vi "Analyze Target.vi"(10 "Goal Pickiness":T1, 11 "Relevant Data":T2[](array[typedef])) -> (3 "What to do":string)   [LabVIEW 2015]
uses:
  References/Relevant Data.ctl
panel:
  in  "Goal Area":dbl
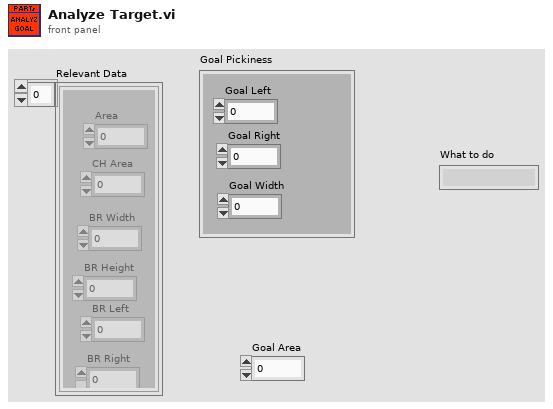
[diagram p1: front panel]
types:
  T1 = cluster{"Goal Left":dbl, "Goal Right":dbl, "Goal Width":dbl}
  T2 = typedef "Relevant Data.ctl" = cluster{"Area":dbl, "CH Area":dbl, "BR Width":dbl, "BR Height":dbl, "BR Left":dbl, "BR Right":dbl}
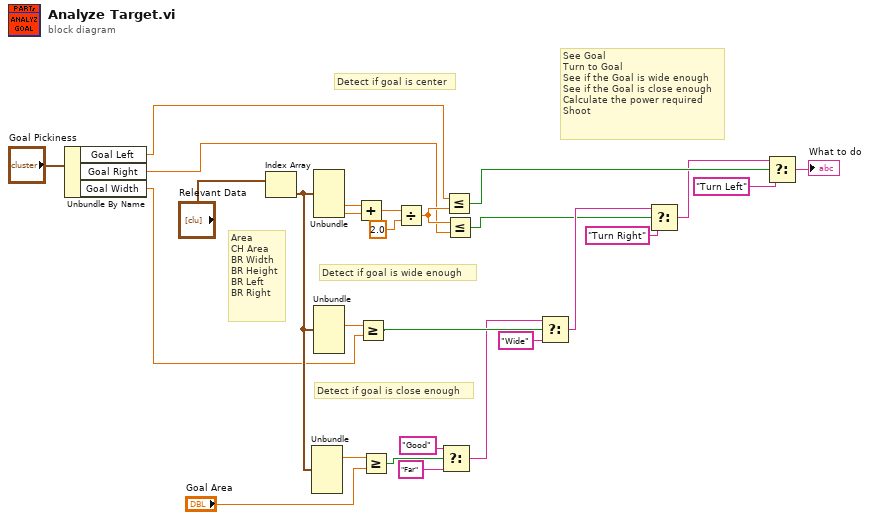
[diagram p0: block diagram]
diagram:
  # "See Goal\nTurn to Goal\nSee if the Goal is wide enough\nSee if the Goal is close enough\nCalculate the power required\nShoot"
  # "Detect if goal is close enough"
  # "Detect if goal is wide enough"
  # "Detect if goal is center"
  # "Area\nCH Area\nBR Width\nBR Height\nBR Left\nBR Right"
  n1 = Unbundle By Name("Goal Pickiness") -> ("Goal Left"=w3:dbl, "Goal Right"=w2:dbl, "Goal Width"=w1:dbl)
  n2 = Index Array(array="Relevant Data") -> (element=w20:T2)  [unwired: 1 in]
  n3 = Unbundle(w20) -> ("CH Area"=w19:dbl)  [unwired: 5 out]
  n4 = Unbundle(w20) -> ("BR Left"=w26:dbl, "BR Right"=w25:dbl)  [unwired: 4 out]
  n5 = Unbundle(w20) -> ("BR Width"=w21:dbl)  [unwired: 5 out]
  n6 = Add(x=w26, y=w25) -> (x+y=w24:dbl)
  n7 = Greater Or Equal?(x=w21, y=w1) -> (x >= y?=w14:bool)
  n8 = Greater Or Equal?(x=w19, y="Goal Area") -> (x >= y?=w18:bool)
  n9 = Divide(x=w24, y=2.0) -> (x/y=w22:dbl)
  n10 = Select(t="Good", s=w18, f="Far") -> (s? t:f=w13:string)
  n11 = Less Or Equal?(x=w3, y=w22) -> (x <= y?=w8:bool)
  n12 = Less Or Equal?(x=w22, y=w2) -> (x <= y?=w9:bool)
  n13 = Select(t=w13, s=w14, f="Wide") -> (s? t:f=w11:string)
  n14 = Select(t=w11, s=w9, f="Turn Right") -> (s? t:f=w7:string)
  n15 = Select(t=w7, s=w8, f="Turn Left") -> (s? t:f=→"What to do":string)
